vi "Read Valve Turbo State.vi"(7 "timeout in ms (-1)":i32, 8 "error in (no error)":errorcluster, 11 "Turbo in":refnum<class "Turbo.lvclass">) -> (0 "error out":errorcluster, 2 "Open?":bool, 3 "Turbo out":refnum<class "Turbo.lvclass">, 4 "Valve Turbo StateQ":refnum<queue>)   [LabVIEW 2015, in "cRIO-Carbondioxide.lvlib" / "CO2-Actor.lvlib" / "Turbo.lvclass"]
uses:
  Turbo.lvclass
  Turbo.lvclass/Turbo.ctl
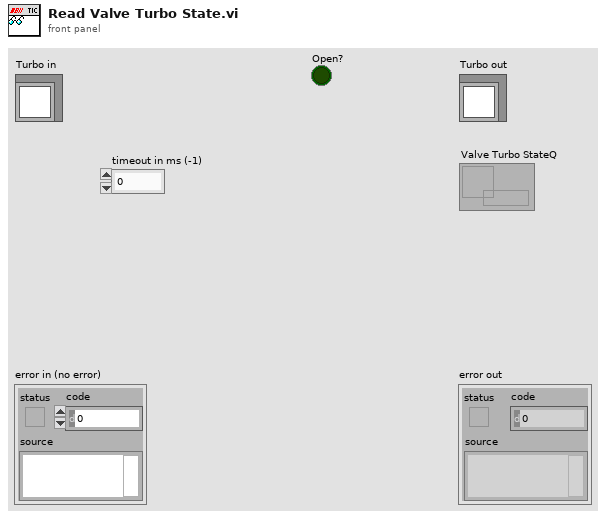
[diagram p1: front panel]
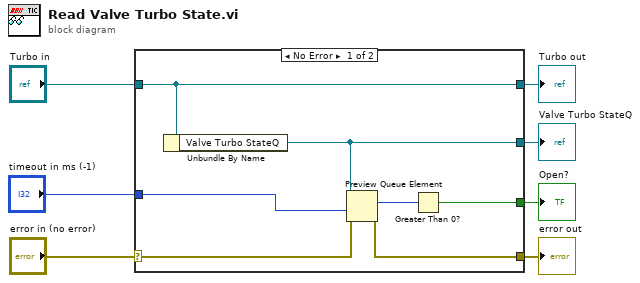
[diagram p0: block diagram]
diagram:
  n1 = case shown="No Error" "error in (no error)" {
    selector: "error in (no error)" -> [w12 w15]
    tunnel: [w11 w15] -> w6
    tunnel: [w14 w16] -> w4
    tunnel: "Turbo in" -> [w14 w16]
    tunnel: [w13 _] -> w3
    tunnel: [w9 _] -> w2
    tunnel: "timeout in ms (-1)" -> [w8 _]
    frame No Error {
      n2 = Unbundle By Name(w14) -> ("Valve Turbo StateQ"=w13:refnum<queue>)
      n3 = Preview Queue Element(queue=w13, timeout in ms (-1)=w8, error in (no error)=w12) -> (element=w10:u16, error out=w11:errorcluster)  [unwired: 2 out]
      n4 = Greater Than 0?(x=w10) -> (x > 0?=w9:bool)
    }
    frame Error {
    }
  }
  "error out" <- w6
  "Turbo out" <- w4
  "Valve Turbo StateQ" <- w3
  "Open?" <- w2
